vi "APC_9049_RT_main.vi"   [LabVIEW 2020]
panel:
  # "monarch APC v0.1"
  # "cRIO 9049 RT main"
types:
  T1 = typedef "APC_DAQqueues.ctl" = cluster{"SignalList":cluster{"CAS":string[], "CycAvg":string[]}, "Queues":cluster{"CAS":refnum<queue>, "CycAvg":refnum<queue>}, "scaled units":string[]}
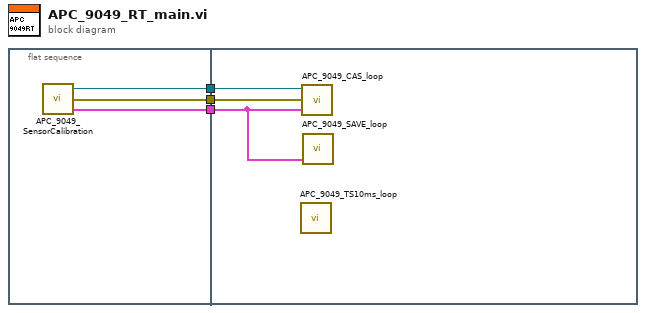
[diagram p0: block diagram]
diagram:
  n1 = flat-sequence {
    tunnel: [w6] -> w3
    tunnel: [w5] -> w2
    tunnel: [w4] -> w1
    tunnel: w3 -> [w9]
    tunnel: w2 -> [w8]
    tunnel: w1 -> [w7]
    frame #0 {
      n2 = call "APC_9049_SensorCalibration.vi"() -> ("DAQqueues"=w4:T1, "error out"=w5:errorcluster, "scaled dAQmx task"=w6:refnum<k21>)
    }
    frame #1 {
      n3 = call "APC_9049_TS10ms_loop.vi"() -> ()  [unwired: 3 in]
      n4 = call "APC_9049_CAS_loop.vi"("DAQqueues"=w7, "error in"=w8, "scaled dAQmx task"=w9) -> ()
      n5 = call "APC_9049_SAVE_loop.vi"("DAQqueues"=w7) -> ()  [unwired: 2 in]
    }
  }
